vi "Test Process No Process Warnings Through Basic Lifecycle.vi"(8 "error in (no error)":errorcluster, 11 "Process Test In":refnum<class "Process Test.lvclass">) -> (0 "error out":errorcluster, 3 "Process Test Out":refnum<class "Process Test.lvclass">)   [LabVIEW 2020, in "Process Test.lvclass"]
uses:
  Process Test.lvclass
  C:/Program Files (x86)/National Instruments/LabVIEW 2020/vi.lib/Asteme/LUnit/Test Case.lvclass
  Mock Error Handler/Mock Error Handler.lvclass
  C:/Users/anton/Documents/GitHub/Triarc-Framework/source/Framework/Error Handler Interface/Error Handler Interface.lvclass
  Framework/Process/Process.lvclass/Process.ctl
  <vilib>/Asteme/LUnit/Test Case.lvclass/Test Case.ctl
  <vilib>/Asteme/LUnit/LUnit Assertion Result.lvclass/LUnit Assertion Result.ctl
  Framework/Process/Protected/Messaging/Enqueue Message.vi
  Framework/Process/Public/Lifecycle/Get Lifecycle State.vi
  Framework/Process/Private/SubVIs/Wait for finish.vi
  Framework/Process/Private/SubVIs/Set Lifecycle State.vi
  <vilib>/Asteme/LUnit/Palette/Fail.vi
  <vilib>/Asteme/LUnit/Palette/Pass.vi
  <vilib>/Asteme/LUnit/Set Assertion Type.vi
  <vilib>/Utility/error.llb/Clear Errors.vi
  <vilib>/Asteme/LUnit/Add test result.vi
  <vilib>/Asteme/LUnit/LUnit Write Passed.vi
  <vilib>/Asteme/LUnit/LUnit Get Test Case.vi
  <vilib>/Asteme/LUnit/Assertion Result/LUnit Get Test Name.vi
  <vilib>/Asteme/LUnit/LUnit Write Message.vi
  <vilib>/Asteme/LUnit/LUnit Write Description.vi
  <vilib>/Asteme/LUnit/LUnit Write Assertion Type.vi
  <vilib>/Asteme/LUnit/Read Test Case Name.vi
  <vilib>/Utility/error.llb/Error Cluster From Error Code.vi
  <vilib>/Asteme/LUnit/LUnit Assertion Result.lvclass
  Framework/Process/Process.lvclass
  <vilib>/Asteme/LUnit/Test Case.lvclass
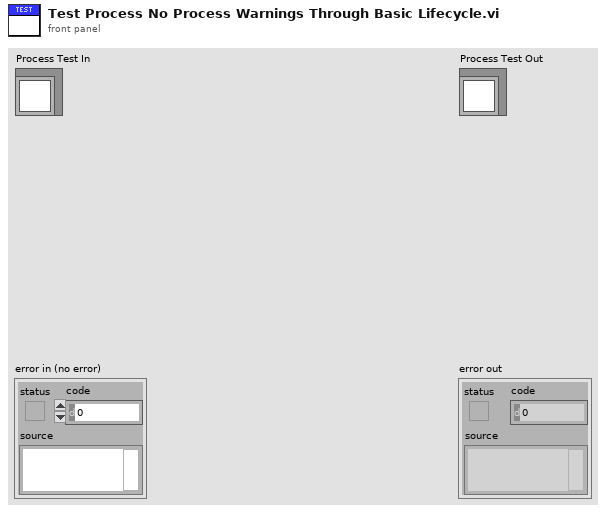
[diagram p1: front panel]
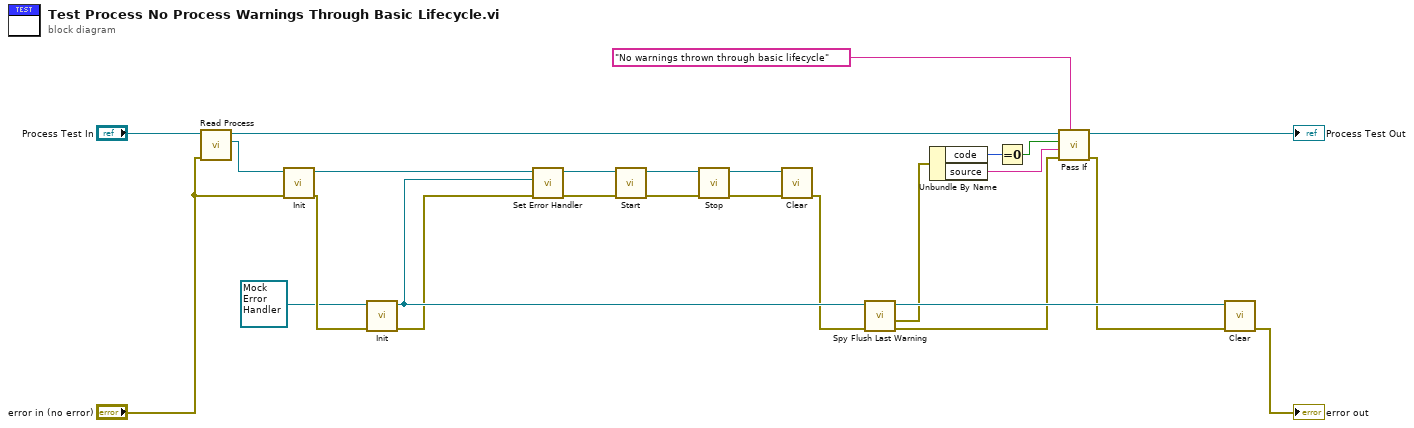
[diagram p0: block diagram]
diagram:
  n1 = call "Read Process.vi"("error in (no error)"="error in (no error)", "Process Test in"="Process Test In") -> ("Process.lvclass"=w8:refnum<class "Process.lvclass">, "Process Test out"=w7:refnum<class "Process Test.lvclass">)  [unwired: 7 in, 1 out]
  n2 = call-dynamic "Init.vi"("error in (no error)"="error in (no error)", "Process In"=w8) -> ("error out"=w25:errorcluster, "Process Out"=w23:refnum<class "Process.lvclass">)  [unwired: 8 in]
  n3 = call-dynamic "Init.vi"("error in (no error)"=w25, "Mock Error Handler In"=refnum<class "Mock Error Handler.lvclass"> refnum ("Mock Error Handler.lvclass")) -> ("error out"=w15:errorcluster, "Mock Error Handler Out"=w16:refnum<class "Mock Error Handler.lvclass">)  [unwired: 8 in]
  n4 = call "Set Error Handler.vi"("error in (no error)"=w15, "Error Handler"=w16, "Process In"=w23) -> ("error out"=w21:errorcluster, "Process Out"=w22:refnum<class "Process.lvclass">)  [unwired: 7 in]
  n5 = call "Start.vi"("error in (no error)"=w21, "Process In"=w22) -> ("error out"=w19:errorcluster, "Process Out"=w20:refnum<class "Process.lvclass">)  [unwired: 8 in]
  n6 = call "Stop.vi"("error in (no error)"=w19, "Process In"=w20) -> ("error out"=w17:errorcluster, "Process Out"=w18:refnum<class "Process.lvclass">)  [unwired: 7 in, 1 out]
  n7 = call-dynamic "Clear.vi"("error in (no error)"=w17, "Process In"=w18) -> ("error out"=w12:errorcluster)  [unwired: 9 in]
  n8 = call "Spy Flush Last Warning.vi"("error in (no error)"=w12, "Mock Error Handler In"=w16) -> ("error out"=w11:errorcluster, "Error"=w4:errorcluster, "Mock Error Handler Out"=w14:refnum<class "Mock Error Handler.lvclass">)  [unwired: 7 in]
  n9 = Unbundle By Name(w4) -> ("code"=w3:i32, "source"=w1:string)
  n10 = Equal To 0?(x=w3) -> (x = 0?=w2:bool)
  n11 = call <vilib>:"Pass If.vi"("Description"="No warnings thrown through basic lifecycle", "error in (no error)"=w11, "Message"=w1, "Pass?"=w2, "Test Case In"=w7) -> ("error out"=w10:errorcluster, "Test Case Out"=→"Process Test Out":refnum<class "Process Test.lvclass">)  [unwired: 5 in]
  n12 = call-dynamic "Clear.vi"("error in (no error)"=w10, "Mock Process In"=w14) -> ("error out"=→"error out":errorcluster)  [unwired: 9 in]
